vi "MarvinTester.vi"() -> ()   [LabVIEW 2017]
uses:
  <vilib>/Instr/_visa.llb/VISA Configure Serial Port (Instr).vi
panel:
  out "TX":string
  out "RX":string
  out "(hi.lo)":u32 format="%.0x"
  in  "GetOUTIO3":bool
  out "S2 GIO 19":bool
  out "S2 GIO 18":bool
  out "S2 GIO 17":bool
  out "S2 GIO 11":bool
  out "S2 GIO 3":bool
  out "S2 GIO 1":bool
  out "S1 GIO 19":bool
  out "S1 GIO 18":bool
  out "S1 GIO 17":bool
  out "S1 GIO 15":bool
  out "S1 GIO 11":bool
  out "S1 GIO 3":bool
  out "S1 GIO 1":bool
  in  "GetIO 2":bool
  out "S2 GIO 15 R":bool
  in  "Reset":bool
  in  "SetDefault":bool
  out "GetIO":u8[](array[numeric])
  out "Ver":string=" "
  in  "Get  ver":bool
  out "PWM Reading":u32
  out "Time Plot":i32=-1
  out "error out":errorcluster
  in  "stop":bool
  in  "Ring":u16(ring) items=["None", "Moment", "Get IO"]
  out "packet PWM":u8[](array[numeric])
  in  "Tab Control":enum32{"Page 3", "Page 4", "Page 2"}(tab)
  in  "GetIO2":bool
  out "out_io1":u32 format="%.0b"
  in  "SetDAC":bool
  in  "I_O":u32 format="%.0b"
  in  "ADC":bool
  in  "ADC num":u8=3
  out "out_io1 2":u32
  in  "DAC":u32
  out "x*y":dbl
  in  "GetADCTester":T1(ring)
  in  "TimeToGet":i32
  in  "Read On/Off":bool
  out "ADCValOutput Single":dbl
  in  "idx":i32
  in  "TA[idx]":bool
  in  "Disconect 2":bool
  in  "110":bool
  in  "120":bool
  in  "90":bool
  in  "60":bool
  in  "100":bool
  in  "20":bool
  in  "70":bool
  in  "40":bool
  in  "30":bool
  in  "80":bool
  in  "50":bool
  in  "10":bool
  in  "25":bool
  in  "0":bool
  in  "COM Port Marvin":refnum<visa-resource-name>="COM1"
  in  "Connect Marvin":bool
  out "CommIcon Marvin":bool=TRUE
  out "String":string
  in  "K15":bool
  in  "Firmeware":bool
  in  "K16":bool
  in  "K17":bool
  in  "Power":bool
  in  "Fan":bool
  in  "VEnable":bool
  out "CurrSp Graph":cluster{"n":dbl, "T":dbl}[](graph)
  out "Frequency":dbl
  in  "Plot On":bool
  in  "Plot OFF":bool
  in  "Get":bool
  in  "Clear":bool
  in  "Plot Time":i32=70
  out "Load":dbl
  out "String 2":string
  in  "COM Port Control":refnum<visa-resource-name>="COM1"
  in  "Time":i32=-1
  out "err tx":errorcluster
  out "Write array":u8[](array[numeric]) format="%x"
  in  "Flag Stop T":bool
  out "VISA":refnum<visa-resource-name>
  out "CommIcon":bool=TRUE
  out "Read array":u8[](array[numeric]) format="%x"
  out "Cmd Id":u8
  in  "Flag Stop I":bool=TRUE
  out "Int b":i32
  in  "Flag Stop R":bool
  out "TX":bool
  out "RX":bool
  in  "Command Menu 2":u16(ring) items=["Status", "Moment", "Isc threshold", "Vin Vout", "RESET FF", "Open", "Close", "Up Time", "Interval Period", "Nm Of Retries", "On time", "Save Parameters", "Version", "Temperature"]
  out "packet":u8[](array[numeric])
  in  "Isc1":i8
  in  "Add Unit":u8
  in  "Disconect":bool
  in  "Connect":bool
  in  "Stop VI":bool
  out "status":bool
  # "Marvin Tester"
  # "[Hz]"
  # "SW Version"
  # "ver : 00.02.a"
  # "I/O"
  # "ADC"
  # "DAC"
  # "0-4"
  # "V=ADC*3.3/4096"
  # "Term1  -0\nTerm2  -1\nCurr   - 2\nEBAYFAN -3\nTempCPU -4"
  # "b0-Rly1\nb1-Rly2\nb2-Rly3\n....\nb20-Rly20\nb21-Power"
  # "[kHz]"
  # "[N.m]"
  # "[msec]"
  # "ver 0.0.1"
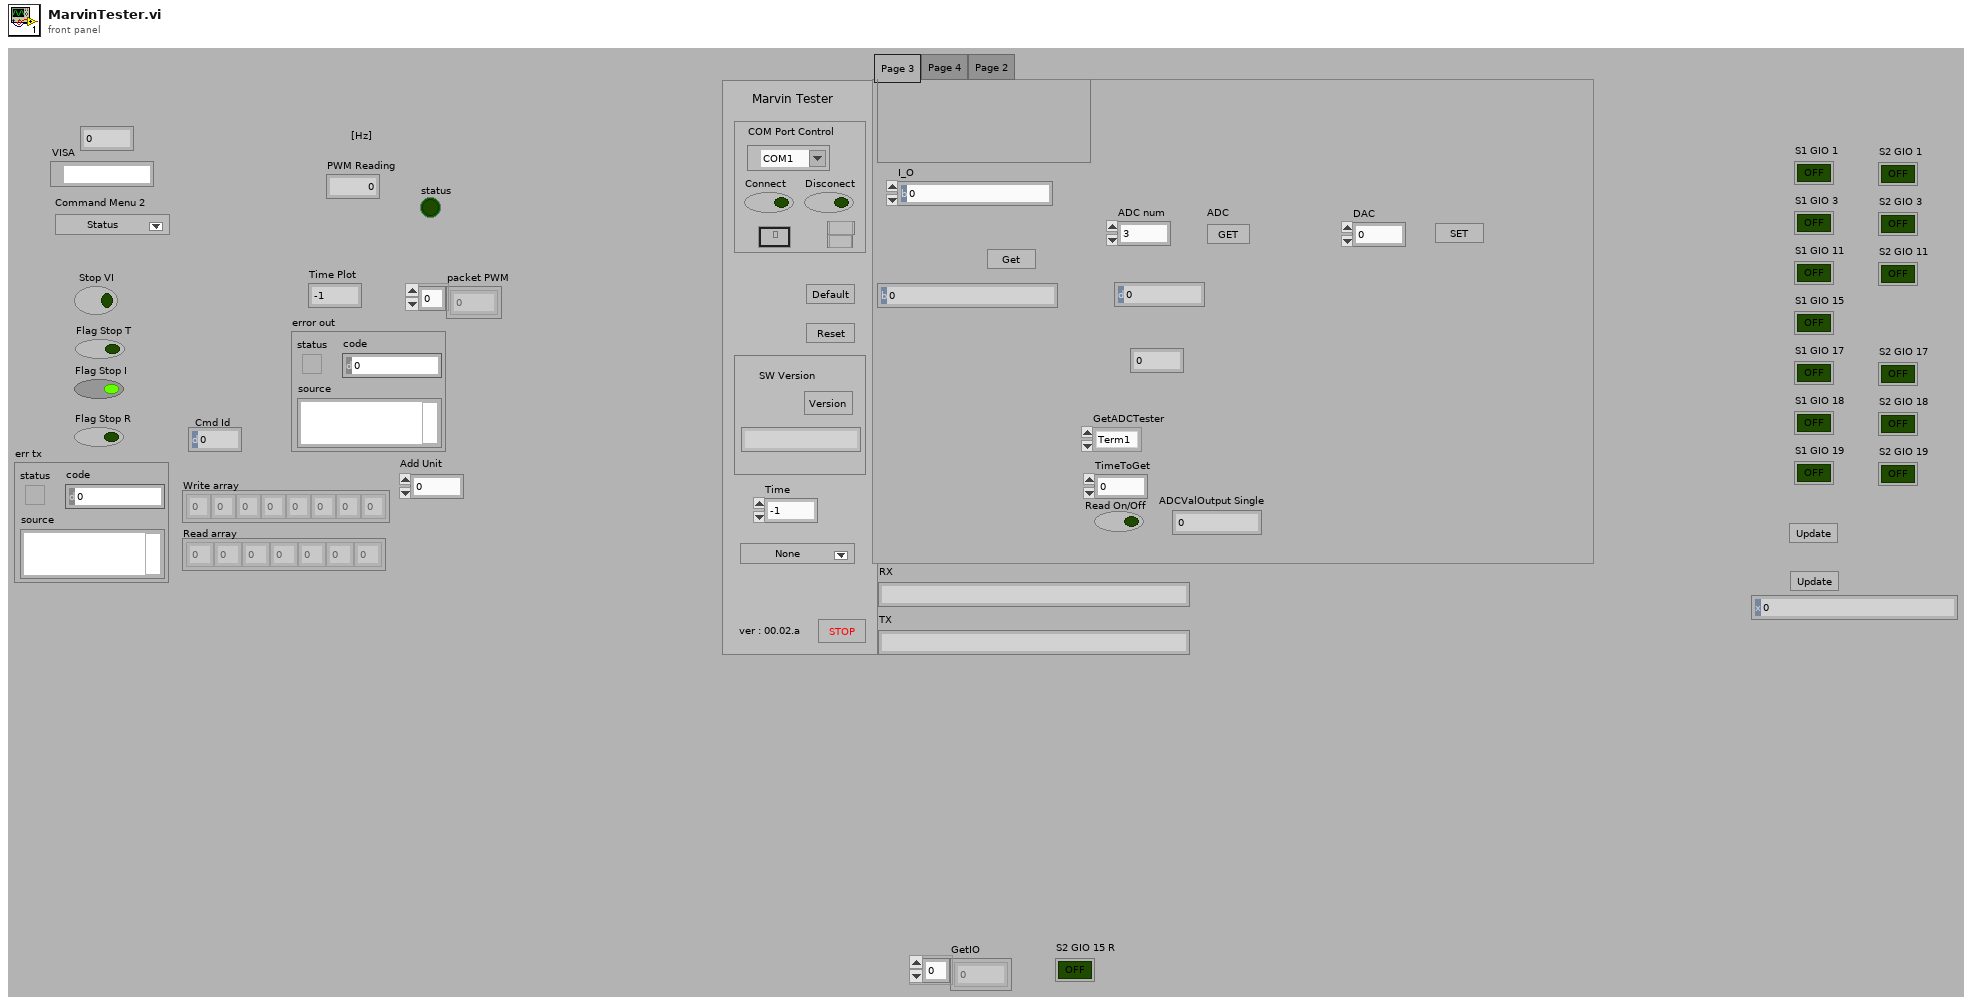
[diagram p1: front panel]
types:
  T1 = enum8{"Term1", "Term2", "Current", "Fan", "TempCPU"}
  T2 = cluster{"d1":dbl, "d2":dbl, "d3":dbl, "id":u16, "d4":dbl}
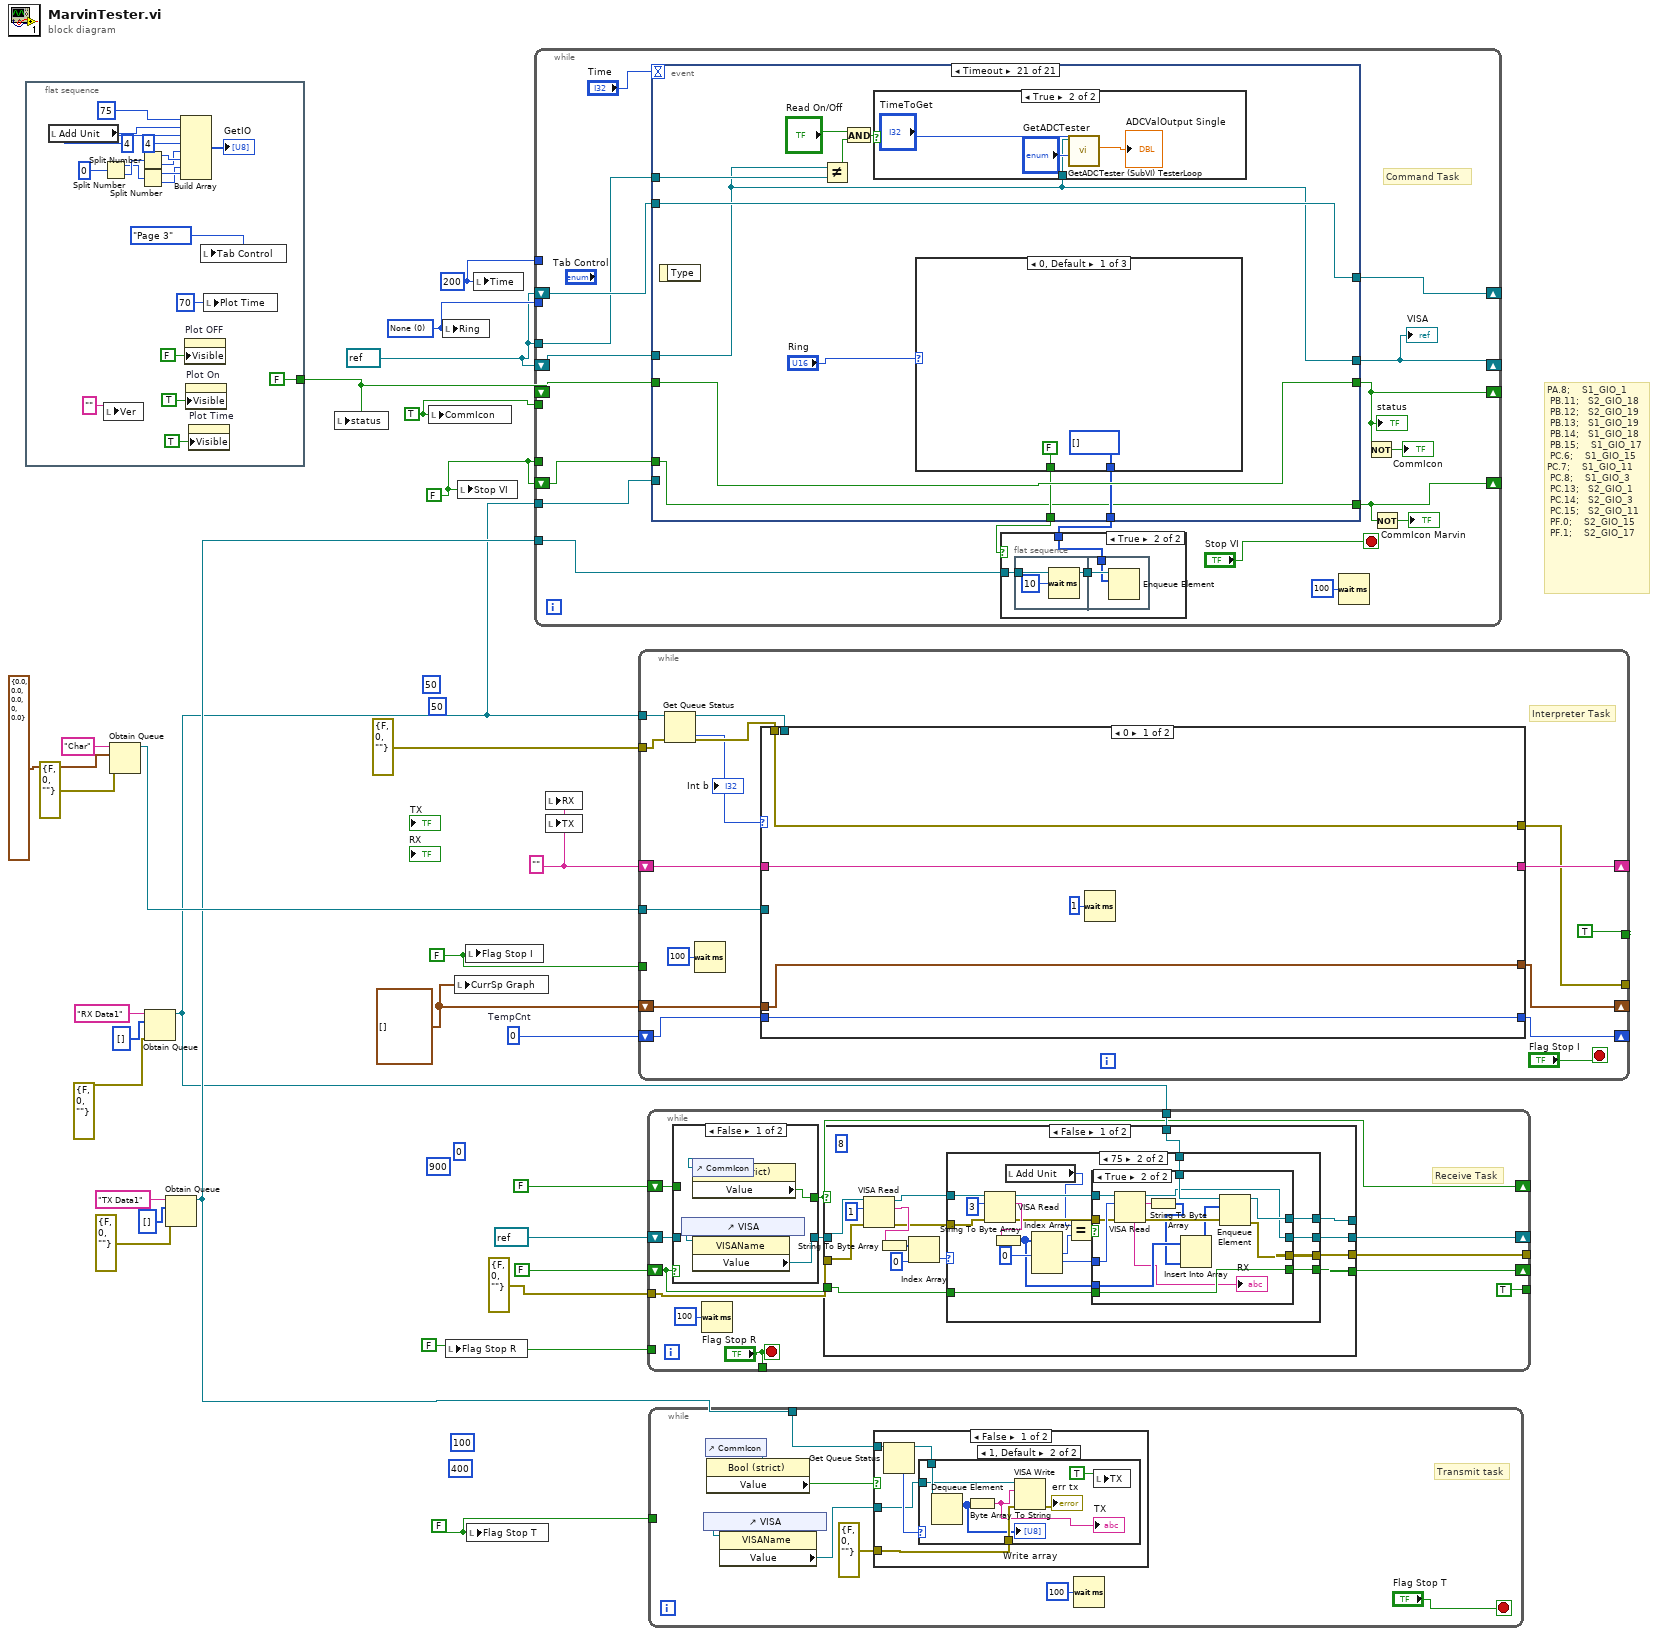
[diagram p0: block diagram]
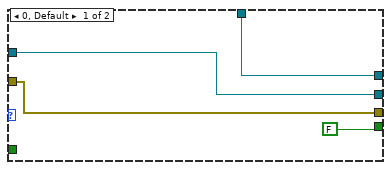
[diagram p3: hidden frame]
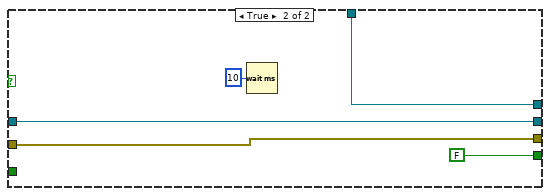
[diagram p5: hidden frame]
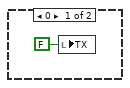
[diagram p6: hidden frame]
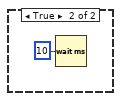
[diagram p7: hidden frame]
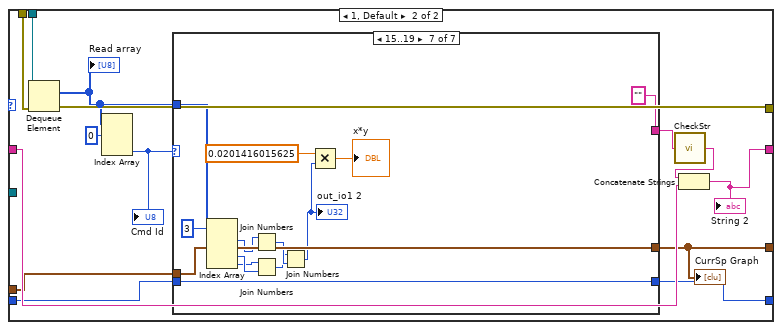
[diagram p8: hidden frame]
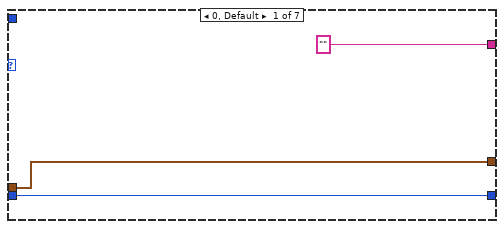
[diagram p9: hidden frame]
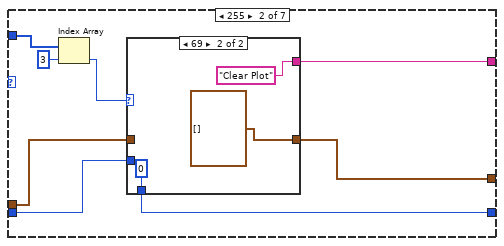
[diagram p10: hidden frame]
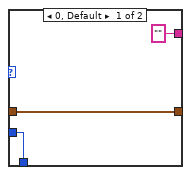
[diagram p11: hidden frame]
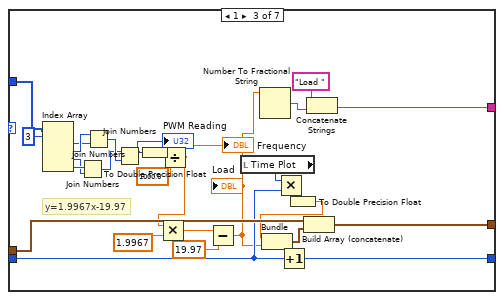
[diagram p12: hidden frame]
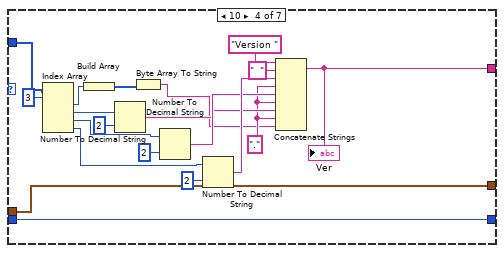
[diagram p13: hidden frame]
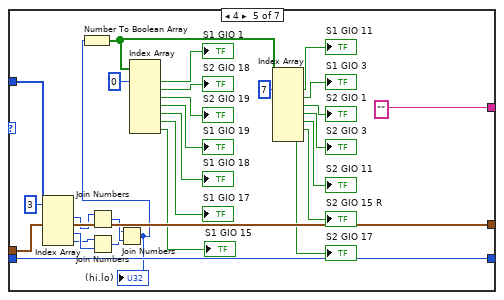
[diagram p14: hidden frame]
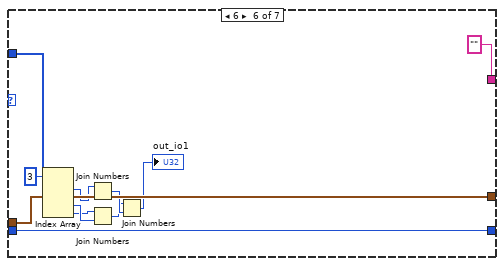
[diagram p15: hidden frame]
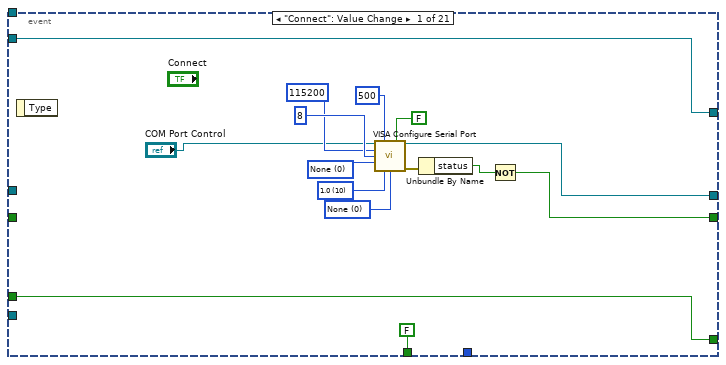
[diagram p17: hidden frame]
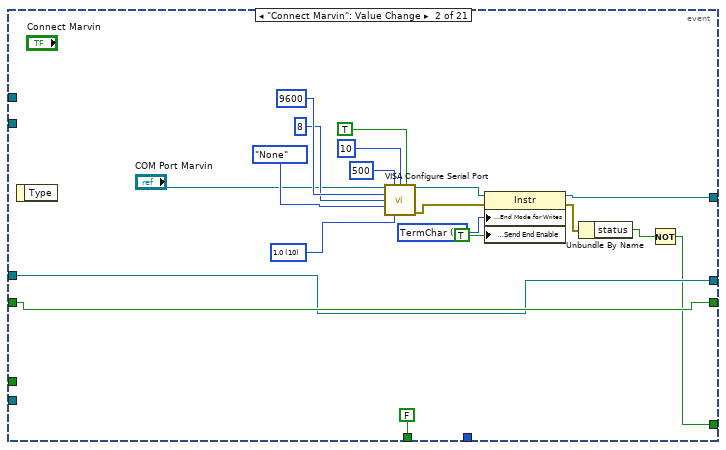
[diagram p18: hidden frame]
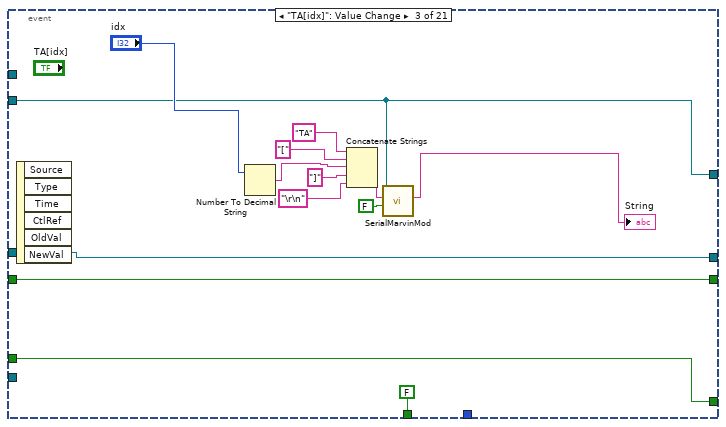
[diagram p19: hidden frame]
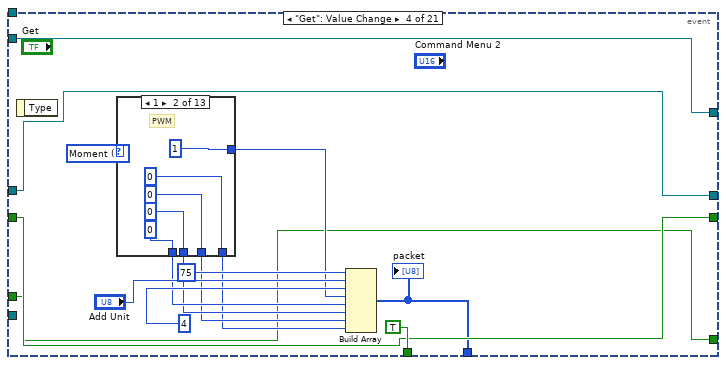
[diagram p20: hidden frame]
diagram:
  w8 = u16 0  # TempCnt
  w5 = cluster{"n":dbl, "T":dbl}[] [] ("Current Graph 4")
  w9 = 200 ("Time")
  w10 = u16 0 items=["None", "Moment"] ("Ring")
  w11 = TRUE ("CommIcon")
  w3 = FALSE
  (unwired) 400 ("Priority")
  (unwired) i64 100 ("Period")
  (unwired) i64 50 ("Period")
  (unwired) 50 ("Priority")
  (unwired) 900 ("Priority")
  (unwired) i64 0 ("Period")
  w14 = FALSE
  w2 = ""
  w28 = FALSE
  w29 = FALSE
  w1 = refnum<visa-resource-name> refnum ("VISA resource name out")
  # "PA.8;   \tS1_GIO_1\n\tPB.11;  \tS2_GIO_18\n\tPB.12;  \tS2_GIO_19\n\tPB.13;  \tS1_GIO_19\n\tPB.14;  \tS1_GIO_18\n\tPB.15;   \tS1_GIO_17\n\tPC.6;   \tS1_GIO_15\nPC.7;   \tS1_GIO_11\n\tPC.8;   \tS1_GIO_3\n\tPC.13;  \tS2_GIO_1\n\tPC.14;  \tS2_GIO_3\n\tPC.15;  \tS2_GIO_11\n\tPF.0;  \t\tS2_GIO_15\n\tPF.1;  \t\tS2_GIO_17"
  n1 = flat-sequence {
    tunnel: [FALSE] -> w7
    frame #0 {
      n2 = local read "Add Unit"() -> (w39:u8)
      n3 = Split Number(x=u32 0) -> (hi(x)=w37:u16, lo(x)=w38:u16)
      n4 = local write "Ver"("" ("Ver")) -> ()
      n5 = Split Number(x=w38) -> (hi(x)=w36:u8, lo(x)=w35:u8)
      n6 = Split Number(x=w37) -> (hi(x)=w34:u8, lo(x)=w33:u8)
      n7 = Build Array(u8 75, w39, u8 4 ("Length"), u8 4, w35, w36, w33, w34) -> (→"GetIO":u8[])
      n8 = property on="Plot OFF" class="Bool"("Visible"=FALSE) -> ()  [unwired: 2 in, 2 out]
      n9 = property on="Plot On" class="Bool"("Visible"=TRUE) -> ()  [unwired: 2 in, 2 out]
      n10 = property on="Plot Time" class="DigNum (strict)"("Visible"=TRUE) -> ()  [unwired: 2 in, 2 out]
      n11 = local write "Tab Control"(enum32{"Page 3", "Page 4", "Page 2"}."Page 3" ("Tab Control")) -> ()
      n12 = local write "Plot Time"(70 ("Plot Time")) -> ()
    }
  }
  n13 = Obtain Queue(name (unnamed)="Char", element data type=T2 {"d1"=0.0, "d2"=0.0, "d3"=0.0, "id"=0, "d4"=0.0}, error in (no error)=errorcluster {"status"=FALSE, "code"=0, "source"=""}) -> (queue out=w19:refnum<queue>)  [unwired: 2 in, 2 out]
  n14 = Obtain Queue(name (unnamed)="RX Data1", element data type=u8[] [], error in (no error)=errorcluster {"status"=FALSE, "code"=0, "source"=""}) -> (queue out=w6:refnum<queue>)  [unwired: 2 in, 2 out]
  n15 = Obtain Queue(name (unnamed)="TX Data1", element data type=u8[] [], error in (no error)=errorcluster {"status"=FALSE, "code"=0, "source"=""}) -> (queue out=w13:refnum<queue>)  [unwired: 2 in, 2 out]
  n16 = local write "status"(w7) -> ()
  n17 = local write "CommIcon"(w11) -> ()
  n18 = local write "Ring"(w10) -> ()
  n19 = local write "Flag Stop R"(w29) -> ()
  n20 = local write "CurrSp Graph"(w5) -> ()
  n21 = local write "Stop VI"(w3) -> ()
  n22 = local write "Flag Stop I"(w28) -> ()
  n23 = local write "Flag Stop T"(w14) -> ()
  n24 = local write "Time"(w9) -> ()
  n25 = while {
    shift-right: [w59] -> _
    shift-left: w1 -> [w66]
    shift-right: [w58] -> _
    shift-left: w7 -> [w65]
    tunnel: w13 -> [w61]
    tunnel: w3 -> [_]
    tunnel: w11 -> [_]
    tunnel: w10 -> [_]
    tunnel: w9 -> [_]
    tunnel: w6 -> [w56]
    shift-right: [w54] -> _
    shift-left: w1 -> [w53]
    shift-right: [w52] -> _
    shift-left: w3 -> [w51]
    tunnel: w1 -> [w50]
    stop <- "Stop VI" stop-if-true
    # "Command Task"
    n26 = event shown="[20] Timeout" {
      selector: _ -> [_ _ _ _ _ _ _ _ _ _ _ _ _ _ _ _ _ _ _ _ _]
      dyn-events: _ -> [_ _ _ _ _ _ _ _ _ _ _ _ _ _ _ _ _ _ _ _ _]
      timeout: "Time" -> [_ _ _ _ _ _ _ _ _ _ _ _ _ _ _ _ _ _ _ _ _]
      tunnel: [w82 w105 w111 w126 w208 w286 w317 w594 w605 w622 w639 w656 w673 w690 w719 w729 w736 w740 refnum<visa-resource-name> refnum ("VISA resource name out") w755 w759] -> w59
      tunnel: w66 -> [_ w105 w111 w126 w208 w286 w317 w594 w605 w622 w639 w656 w673 w690 w719 w729 w736 w740 w751 w755 w759]
      tunnel: [w80 w106 w110 w125 w207 w296 w316 w597 w613 w630 w647 w664 w681 w698 w721 w731 w738 FALSE FALSE w753 w768] -> w58
      tunnel: w65 -> [_ w106 w110 w125 w207 w296 w316 w597 w613 w630 w647 w664 w681 w698 w721 w731 w738 _ _ w753 w768]
      tunnel: [_ _ _ w124 w206 w295 w319 w596 w603 w620 w637 w654 w671 w688 _ _ _ _ _ _ w766] -> w60
      tunnel: [FALSE FALSE FALSE TRUE TRUE TRUE TRUE TRUE TRUE TRUE TRUE TRUE TRUE TRUE FALSE FALSE FALSE FALSE FALSE FALSE w767] -> w62
      tunnel: w56 -> [_ _ _ _ _ _ _ _ _ _ _ _ _ _ _ _ w735 _ _ _ _]
      tunnel: [w75 w92 w112 w123 w203 w284 w315 w589 w602 w619 w636 w653 w670 w687 w704 w723 w733 w741 w747 refnum<visa-resource-name> refnum ("VISA resource name out") w764] -> w54
      tunnel: w53 -> [w75 _ w112 w123 w203 w284 w315 w589 w602 w619 w636 w653 w670 w687 w704 w723 w733 w741 w747 w754 w764]
      tunnel: [w74 w89 w108 w122 w202 w283 w314 w588 w601 w618 w635 w652 w669 w686 w703 w722 w732 w739 w746 FALSE w763] -> w52
      tunnel: w51 -> [w74 _ w108 w122 w202 w283 w314 w588 w601 w618 w635 w652 w669 w686 w703 w722 w732 w739 w746 _ w763]
      tunnel: w50 -> [_ _ _ _ _ _ _ _ _ _ _ _ _ _ _ _ _ _ _ _ w760]
      event "Connect": Value Change {
        w88 = u16 0 items=["None"=0, "XON/XOFF"=1, "RTS/CTS"=2, "DTR/DSR"=4] ("flow control")
        w87 = u16 10 items=["1.0"=10, "1.5"=15, "2.0"=20] ("stop bits")
        w86 = u16 0 items=["None", "Odd", "Even", "Mark", "Space"] ("parity")
        n27 = event-data() -> ()  [unwired: 1 in, 1 out]
        n28 = call-poly "VISA Configure Serial Port"("VISA resource name"="COM Port Control", "timeout (10sec)"=u32 500, "Enable Termination\nChar (T)"=FALSE ("Enable Termination\nChar (T)"), "baud rate (9600)"=u32 115200 ("baud rate"), "data bits (8)"=u16 8 ("data bits"), "parity (0:none)"=w86, "stop bits (10: 1 bit)"=w87, "flow control (0:none)"=w88) -> ("VISA resource name out"=w82:refnum<visa-resource-name>, "error out"=w79:errorcluster)  [unwired: 6 in]
        n29 = Unbundle By Name(w79) -> ("status"=w81:bool)
        n30 = Not(x=w81) -> (.not. x?=w80:bool)
      }
      event "Connect Marvin": Value Change {
        w104 = u16 2 items=["None", "LastBit", "TermChar", "Break"] ("Serial Settings:Serial End Mode for Writes")
        w97 = u16 10 items=["1.0"=10, "1.5"=15, "2.0"=20] ("stop bits (10: 1 bit)")
        n31 = event-data() -> ()  [unwired: 1 in, 1 out]
        n32 = call-poly "VISA Configure Serial Port"("VISA resource name"="COM Port Marvin", "timeout (10sec)"=u32 500, "termination char\n(0xA = '\\n' = LF)"=u8 10 ("termination char\n(0xA = '\\n' = LF)"), "Enable Termination\nChar (T)"=TRUE ("Enable Termination\nChar (T)"), "baud rate (9600)"=u32 9600, "data bits (8)"=u16 8, "parity (0:none)"=enum16{"None", "Odd", "Even", "Mark", "Space"}."None", "stop bits (10: 1 bit)"=w97) -> ("VISA resource name out"=w95:refnum<visa-resource-name>, "error out"=w94:errorcluster)  [unwired: 6 in]
        n33 = property class="Instr"(reference=w95, error in=w94, "Serial Settings:End Mode for Writes"=w104, "Message Based Settings:Send End Enable"=TRUE) -> (reference out=w92:refnum<visa-resource-name>, error out=w90:errorcluster)
        n34 = Unbundle By Name(w90) -> ("status"=w91:bool)
        n35 = Not(x=w91) -> (.not. x?=w89:bool)
      }
      event "TA[idx]": Value Change {
        n36 = event-data() -> ()  [unwired: 1 in, 6 out]
        n37 = Number To Decimal String(number="idx") -> (decimal integer string=w115:string)  [unwired: 1 in]
        n38 = Concatenate Strings("TA" ("string"), "[", w115, "]", "\r\n" ("write buffer")) -> (w116:string)
        n39 = call "SerialMarvinMod.vi"("Clear Log"=FALSE, "write buffer"=w116, "VISA resource name"=w112) -> ("read buffer"=→"String":string)  [unwired: 7 in, 1 out]
      }
      event "Get": Value Change {
        w128 = u16 1 items=["Status", "Moment", "Isc threshold", "Vin Vout", "RESET FF", "Open", "Close", "Up Time", "Interval Period", "Nm Of Retries", "On time", "Save Parameters", "Version", "Temperature"] ("Command Menu 3")
        n40 = event-data() -> ()  [unwired: 1 in, 1 out]
        n41 = case shown="1" w128 {
          tunnel: [u8 0 u8 1 u8 2 u8 15 u8 4 u8 4 u8 5 u8 6 u8 7 u8 8 u8 9 u8 10 u8 16] -> w133
          tunnel: [u8 0 u8 0 u8 0 u8 0 u8 0 u8 0 u8 0 u8 0 u8 0 u8 0 u8 0 u8 0 u8 0] -> w131
          tunnel: [u8 0 u8 0 u8 0 u8 0 u8 0 u8 0 u8 0 u8 0 u8 0 u8 0 u8 0 u8 0 u8 0] -> w130
          tunnel: [u8 0 u8 0 "Isc1" u8 0 u8 1 u8 0 u8 0 u8 0 u8 0 u8 0 u8 0 u8 0 u8 0] -> w132
          tunnel: [u8 0 u8 0 u8 0 u8 0 u8 0 u8 0 u8 0 u8 0 u8 0 u8 0 u8 0 u8 0 u8 0] -> w129
          frame 0, Default {
            # "Status"
          }
          frame 1 {
            # "PWM"
          }
          frame 2 {
          }
          frame 3 {
            # "Vout"
          }
          frame 5 {
          }
          frame 6 {
          }
          frame 7 {
          }
          frame 8 {
          }
          frame 9 {
          }
          frame 10 {
          }
          frame 11 {
          }
          frame 12 {
          }
          frame 13 {
          }
        }
        n42 = Build Array(u8 75, "Add Unit", u8 4 ("Length"), w133, w132, w131, w130, w129) -> (w124:u8[])
        "packet" <- w124
      }
      event "Get  ver": Value Change {
        w210 = u16 12 items=["Status", "Moment", "Isc threshold", "Vin Vout", "RESET FF", "Open", "Close", "Up Time", "Interval Period", "Nm Of Retries", "On time", "Save Parameters", "Version", "Temperature"] ("Command Menu 3")
        n43 = event-data() -> ()  [unwired: 1 in, 1 out]
        n44 = local read "Add Unit"() -> (w205:u8)
        n45 = case shown="0, Default" w210 {
          tunnel: [u8 0 u8 1 u8 2 u8 15 u8 4 u8 4 u8 5 u8 6 u8 7 u8 8 u8 9 u8 10 u8 16] -> w215
          tunnel: [u8 0 u8 0 u8 0 u8 0 u8 0 u8 0 u8 0 u8 0 u8 0 u8 0 u8 0 u8 0 u8 0] -> w213
          tunnel: [u8 0 u8 0 u8 0 u8 0 u8 0 u8 0 u8 0 u8 0 u8 0 u8 0 u8 0 u8 0 u8 0] -> w212
          tunnel: [u8 0 u8 0 u8 0 u8 0 u8 1 u8 0 u8 0 u8 0 u8 0 u8 0 u8 0 u8 0 u8 0] -> w214
          tunnel: [u8 0 u8 0 u8 0 u8 0 u8 0 u8 0 u8 0 u8 0 u8 0 u8 0 u8 0 u8 0 u8 0] -> w211
          frame 0, Default {
            # "Status"
          }
          frame 1 {
            # "PWM"
          }
          frame 2 {
          }
          frame 3 {
            # "Vout"
          }
          frame 5 {
          }
          frame 6 {
          }
          frame 7 {
          }
          frame 8 {
          }
          frame 9 {
          }
          frame 10 {
          }
          frame 11 {
          }
          frame 12 {
          }
          frame 13 {
          }
        }
        n46 = local write "Ver"("" ("Ver")) -> ()
        n47 = Build Array(u8 75, w205, u8 4 ("Length"), w215, w214, w213, w212, w211) -> (w206:u8[])
      }
      event "I_O": Value Change {
        n48 = event-data() -> ()  [unwired: 1 in, 3 out]
        n49 = local read "Add Unit"() -> (w294:u8)
        n50 = To Unsigned Long Integer(number="I_O") -> (unsigned 32bit integer=w287:u32)
        n51 = Split Number(x=w287) -> (hi(x)=w292:u16, lo(x)=w293:u16)
        n52 = Split Number(x=w293) -> (hi(x)=w291:u8, lo(x)=w290:u8)
        n53 = Split Number(x=w292) -> (hi(x)=w289:u8, lo(x)=w288:u8)
        n54 = Build Array(u8 75, w294, u8 4 ("Length"), u8 2, w290, w291, w288, w289) -> (w295:u8[])
      }
      event "0", "25", "10", "50", "80", "30", "40", "70", "20", "100", "60", "90", "120", "110", "K15", "Firmeware", "K16", "K17", "Power", "Fan", "VEnable": Value Change {
        n55 = event-data() -> ("CtlRef"=w322:refnum<vi>, "NewVal"=w320:bool)  [unwired: 1 in, 1 out]
        n56 = property class="Bool (strict)"(reference=w322) -> ("Label.Text"=w321:string)  [unwired: 1 in, 2 out]
        n57 = Build Array("K15", "K16", "K17", "VEnable", "Firmeware", "Fan", "Power") -> (w302:bool[])
        n58 = Initialize Array(FALSE, 14 ("dimension size")) -> (w303:bool[])
        n59 = Build Array (concatenate)(w303, w302) -> (w301:bool[])
        n60 = Boolean Array To Number(Boolean array=w301) -> (number=w306:u32)
        n61 = case shown="\"120\"" w321 {
          tunnel: w320 -> [w330 w348 w365 w383 w400 w418 w436 w455 w473 w490 w509 w526 w544 w562 _]
          tunnel: [w327 w345 w362 w380 w397 w415 w433 w452 w470 w487 w506 w523 w541 w559 w575] -> w319
          tunnel: w306 -> [w324 w343 w359 w378 w395 w413 w431 w450 w469 w485 w504 w521 w539 w557 w576]
          frame "0" {
            n62 = Select(t=u32 1 ("number"), s=w330, f=u32 0) -> (s? t:f=w328:u32)
            n63 = local read "Add Unit"() -> (w331:u8)
            n64 = To Unsigned Long Integer(number=w328) -> (unsigned 32bit integer=w325:u32)
            n65 = Or(x=w324, y=w325) -> (x .or. y?=w323:u32)
            n66 = Split Number(x=w323) -> (hi(x)=w336:u16, lo(x)=w337:u16)
            n67 = Split Number(x=w337) -> (hi(x)=w335:u8, lo(x)=w334:u8)
            n68 = Split Number(x=w336) -> (hi(x)=w333:u8, lo(x)=w332:u8)
            n69 = Build Array(u8 75, w331, u8 4 ("Length"), u8 2, w334, w335, w332, w333) -> (w327:u8[])
          }
          frame "10" {
            n70 = Select(t=u32 2 ("number"), s=w348, f=u32 0) -> (s? t:f=w346:u32)
            n71 = local read "Add Unit"() -> (w349:u8)
            n72 = To Unsigned Long Integer(number=w346) -> (unsigned 32bit integer=w342:u32)
            n73 = Or(x=w343, y=w342) -> (x .or. y?=w341:u32)
            n74 = Split Number(x=w341) -> (hi(x)=w354:u16, lo(x)=w355:u16)
            n75 = Split Number(x=w355) -> (hi(x)=w353:u8, lo(x)=w352:u8)
            n76 = Split Number(x=w354) -> (hi(x)=w351:u8, lo(x)=w350:u8)
            n77 = Build Array(u8 75, w349, u8 4 ("Length"), u8 2, w352, w353, w350, w351) -> (w345:u8[])
          }
          frame "20" {
            n78 = Select(t=u32 4 ("number"), s=w365, f=u32 0) -> (s? t:f=w363:u32)
            n79 = local read "Add Unit"() -> (w367:u8)
            n80 = To Unsigned Long Integer(number=w363) -> (unsigned 32bit integer=w361:u32)
            n81 = Or(x=w359, y=w361) -> (x .or. y?=w360:u32)
            n82 = Split Number(x=w360) -> (hi(x)=w372:u16, lo(x)=w373:u16)
            n83 = Split Number(x=w373) -> (hi(x)=w371:u8, lo(x)=w370:u8)
            n84 = Split Number(x=w372) -> (hi(x)=w369:u8, lo(x)=w368:u8)
            n85 = Build Array(u8 75, w367, u8 4 ("Length"), u8 2, w370, w371, w368, w369) -> (w362:u8[])
          }
          frame "25" {
            n86 = Select(t=u32 8 ("number"), s=w383, f=u32 0) -> (s? t:f=w381:u32)
            n87 = local read "Add Unit"() -> (w385:u8)
            n88 = To Unsigned Long Integer(number=w381) -> (unsigned 32bit integer=w379:u32)
            n89 = Or(x=w378, y=w379) -> (x .or. y?=w377:u32)
            n90 = Split Number(x=w377) -> (hi(x)=w390:u16, lo(x)=w391:u16)
            n91 = Split Number(x=w391) -> (hi(x)=w389:u8, lo(x)=w388:u8)
            n92 = Split Number(x=w390) -> (hi(x)=w387:u8, lo(x)=w386:u8)
            n93 = Build Array(u8 75, w385, u8 4 ("Length"), u8 2, w388, w389, w386, w387) -> (w380:u8[])
          }
          frame "30" {
            n94 = Select(t=u32 16 ("number"), s=w400, f=u32 0) -> (s? t:f=w398:u32)
            n95 = local read "Add Unit"() -> (w402:u8)
            n96 = To Unsigned Long Integer(number=w398) -> (unsigned 32bit integer=w403:u32)
            n97 = Or(x=w403, y=w395) -> (x .or. y?=w396:u32)
            n98 = Split Number(x=w396) -> (hi(x)=w408:u16, lo(x)=w409:u16)
            n99 = Split Number(x=w409) -> (hi(x)=w407:u8, lo(x)=w406:u8)
            n100 = Split Number(x=w408) -> (hi(x)=w405:u8, lo(x)=w404:u8)
            n101 = Build Array(u8 75, w402, u8 4 ("Length"), u8 2, w406, w407, w404, w405) -> (w397:u8[])
          }
          frame "40" {
            n102 = Select(t=u32 32 ("number"), s=w418, f=u32 0) -> (s? t:f=w416:u32)
            n103 = local read "Add Unit"() -> (w420:u8)
            n104 = To Unsigned Long Integer(number=w416) -> (unsigned 32bit integer=w421:u32)
            n105 = Or(x=w413, y=w421) -> (x .or. y?=w414:u32)
            n106 = Split Number(x=w414) -> (hi(x)=w426:u16, lo(x)=w427:u16)
            n107 = Split Number(x=w427) -> (hi(x)=w425:u8, lo(x)=w424:u8)
            n108 = Split Number(x=w426) -> (hi(x)=w423:u8, lo(x)=w422:u8)
            n109 = Build Array(u8 75, w420, u8 4 ("Length"), u8 2, w424, w425, w422, w423) -> (w415:u8[])
          }
          frame "50" {
            n110 = Select(t=u32 64 ("number"), s=w436, f=u32 0) -> (s? t:f=w434:u32)
            n111 = local read "Add Unit"() -> (w438:u8)
            n112 = To Unsigned Long Integer(number=w434) -> (unsigned 32bit integer=w439:u32)
            n113 = Or(x=w431, y=w439) -> (x .or. y?=w432:u32)
            n114 = Split Number(x=w432) -> (hi(x)=w444:u16, lo(x)=w445:u16)
            n115 = Split Number(x=w445) -> (hi(x)=w443:u8, lo(x)=w442:u8)
            n116 = Split Number(x=w444) -> (hi(x)=w441:u8, lo(x)=w440:u8)
            n117 = Build Array(u8 75, w438, u8 4 ("Length"), u8 2, w442, w443, w440, w441) -> (w433:u8[])
          }
          frame "60" {
            n118 = Select(t=u32 128 ("number"), s=w455, f=u32 0) -> (s? t:f=w453:u32)
            n119 = local read "Add Unit"() -> (w457:u8)
            n120 = To Unsigned Long Integer(number=w453) -> (unsigned 32bit integer=w451:u32)
            n121 = Or(x=w450, y=w451) -> (x .or. y?=w449:u32)
            n122 = Split Number(x=w449) -> (hi(x)=w462:u16, lo(x)=w463:u16)
            n123 = Split Number(x=w463) -> (hi(x)=w461:u8, lo(x)=w460:u8)
            n124 = Split Number(x=w462) -> (hi(x)=w459:u8, lo(x)=w458:u8)
            n125 = Build Array(u8 75, w457, u8 4 ("Length"), u8 2, w460, w461, w458, w459) -> (w452:u8[])
          }
          frame "70" {
            n126 = Select(t=u32 256 ("number"), s=w473, f=u32 0) -> (s? t:f=w471:u32)
            n127 = local read "Add Unit"() -> (w475:u8)
            n128 = To Unsigned Long Integer(number=w471) -> (unsigned 32bit integer=w468:u32)
            n129 = Or(x=w469, y=w468) -> (x .or. y?=w467:u32)
            n130 = Split Number(x=w467) -> (hi(x)=w480:u16, lo(x)=w481:u16)
            n131 = Split Number(x=w481) -> (hi(x)=w479:u8, lo(x)=w478:u8)
            n132 = Split Number(x=w480) -> (hi(x)=w477:u8, lo(x)=w476:u8)
            n133 = Build Array(u8 75, w475, u8 4 ("Length"), u8 2, w478, w479, w476, w477) -> (w470:u8[])
          }
          frame "80" {
            n134 = Select(t=u32 512 ("number"), s=w490, f=u32 0) -> (s? t:f=w488:u32)
            n135 = local read "Add Unit"() -> (w492:u8)
            n136 = To Unsigned Long Integer(number=w488) -> (unsigned 32bit integer=w493:u32)
            n137 = Or(x=w485, y=w493) -> (x .or. y?=w486:u32)
            n138 = Split Number(x=w486) -> (hi(x)=w498:u16, lo(x)=w499:u16)
            n139 = Split Number(x=w499) -> (hi(x)=w497:u8, lo(x)=w496:u8)
            n140 = Split Number(x=w498) -> (hi(x)=w495:u8, lo(x)=w494:u8)
            n141 = Build Array(u8 75, w492, u8 4 ("Length"), u8 2, w496, w497, w494, w495) -> (w487:u8[])
          }
          frame "90" {
            n142 = Select(t=u32 1024 ("number"), s=w509, f=u32 0) -> (s? t:f=w507:u32)
            n143 = local read "Add Unit"() -> (w511:u8)
            n144 = To Unsigned Long Integer(number=w507) -> (unsigned 32bit integer=w505:u32)
            n145 = Or(x=w504, y=w505) -> (x .or. y?=w503:u32)
            n146 = Split Number(x=w503) -> (hi(x)=w516:u16, lo(x)=w517:u16)
            n147 = Split Number(x=w517) -> (hi(x)=w515:u8, lo(x)=w514:u8)
            n148 = Split Number(x=w516) -> (hi(x)=w513:u8, lo(x)=w512:u8)
            n149 = Build Array(u8 75, w511, u8 4 ("Length"), u8 2, w514, w515, w512, w513) -> (w506:u8[])
          }
          frame "100" {
            n150 = Select(t=u32 2048 ("number"), s=w526, f=u32 0) -> (s? t:f=w524:u32)
            n151 = local read "Add Unit"() -> (w528:u8)
            n152 = To Unsigned Long Integer(number=w524) -> (unsigned 32bit integer=w529:u32)
            n153 = Or(x=w521, y=w529) -> (x .or. y?=w522:u32)
            n154 = Split Number(x=w522) -> (hi(x)=w534:u16, lo(x)=w535:u16)
            n155 = Split Number(x=w535) -> (hi(x)=w533:u8, lo(x)=w532:u8)
            n156 = Split Number(x=w534) -> (hi(x)=w531:u8, lo(x)=w530:u8)
            n157 = Build Array(u8 75, w528, u8 4 ("Length"), u8 2, w532, w533, w530, w531) -> (w523:u8[])
          }
          frame "110" {
            n158 = local read "Add Unit"() -> (w546:u8)
            n159 = Select(t=u32 4096 ("number"), s=w544, f=u32 0) -> (s? t:f=w542:u32)
            n160 = To Unsigned Long Integer(number=w542) -> (unsigned 32bit integer=w547:u32)
            n161 = Or(x=w539, y=w547) -> (x .or. y?=w540:u32)
            n162 = Split Number(x=w540) -> (hi(x)=w552:u16, lo(x)=w553:u16)
            n163 = Split Number(x=w553) -> (hi(x)=w551:u8, lo(x)=w550:u8)
            n164 = Split Number(x=w552) -> (hi(x)=w549:u8, lo(x)=w548:u8)
            n165 = Build Array(u8 75, w546, u8 4 ("Length"), u8 2, w550, w551, w548, w549) -> (w541:u8[])
          }
          frame "120" {
            n166 = Select(t=u32 8192 ("number"), s=w562, f=u32 0) -> (s? t:f=w560:u32)
            n167 = local read "Add Unit"() -> (w564:u8)
            n168 = To Unsigned Long Integer(number=w560) -> (unsigned 32bit integer=w565:u32)
            n169 = Or(x=w565, y=w557) -> (x .or. y?=w558:u32)
            n170 = Split Number(x=w558) -> (hi(x)=w570:u16, lo(x)=w571:u16)
            n171 = Split Number(x=w571) -> (hi(x)=w569:u8, lo(x)=w568:u8)
            n172 = Split Number(x=w570) -> (hi(x)=w567:u8, lo(x)=w566:u8)
            n173 = Build Array(u8 75, w564, u8 4 ("Length"), u8 2, w568, w569, w566, w567) -> (w559:u8[])
          }
          frame Default {
            n174 = local read "Add Unit"() -> (w577:u8)
            n175 = To Unsigned Long Integer(number=w576) -> (unsigned 32bit integer=w578:u32)
            n176 = Split Number(x=w578) -> (hi(x)=w583:u16, lo(x)=w584:u16)
            n177 = Split Number(x=w584) -> (hi(x)=w582:u8, lo(x)=w581:u8)
            n178 = Split Number(x=w583) -> (hi(x)=w580:u8, lo(x)=w579:u8)
            n179 = Build Array(u8 75, w577, u8 4 ("Length"), u8 2, w581, w582, w579, w580) -> (w575:u8[])
          }
        }
      }
      event "ADC": Value Change {
        w590 = u8 0 ("element")
        n180 = event-data() -> ()  [unwired: 1 in, 3 out]
        n181 = local read "Add Unit"() -> (w595:u8)
        n182 = Add(x="ADC num", y=u8 15) -> (x+y=w592:u8)
        n183 = Build Array(u8 75, w595, u8 4 ("Length"), w592, w590, w590, w590, w590) -> (w596:u8[])
      }
      event "GetIO 2": Value Change {
        n184 = event-data() -> ()  [unwired: 1 in, 1 out]
        n185 = local read "Add Unit"() -> (w612:u8)
        n186 = Split Number(x=u32 0) -> (hi(x)=w610:u16, lo(x)=w611:u16)
        n187 = Split Number(x=w611) -> (hi(x)=w609:u8, lo(x)=w608:u8)
        n188 = Split Number(x=w610) -> (hi(x)=w607:u8, lo(x)=w606:u8)
        n189 = Build Array(u8 75, w612, u8 4 ("Length"), u8 4, w608, w609, w606, w607) -> (w603:u8[])
        n190 = local write "GetIO"(w603) -> ()
      }
      event "SetDefault": Value Change {
        n191 = event-data() -> ()  [unwired: 1 in, 1 out]
        n192 = local read "Add Unit"() -> (w629:u8)
        n193 = Split Number(x=u32 0) -> (hi(x)=w627:u16, lo(x)=w628:u16)
        n194 = Split Number(x=w628) -> (hi(x)=w626:u8, lo(x)=w625:u8)
        n195 = Split Number(x=w627) -> (hi(x)=w624:u8, lo(x)=w623:u8)
        n196 = Build Array(u8 75, w629, u8 4 ("Length"), u8 9, w625, w626, w623, w624) -> (w620:u8[])
        n197 = local write "GetIO"(w620) -> ()
      }
      event "Reset": Value Change {
        n198 = event-data() -> ()  [unwired: 1 in, 1 out]
        n199 = local read "Add Unit"() -> (w646:u8)
        n200 = Split Number(x=u32 0) -> (hi(x)=w644:u16, lo(x)=w645:u16)
        n201 = Split Number(x=w645) -> (hi(x)=w643:u8, lo(x)=w642:u8)
        n202 = Split Number(x=w644) -> (hi(x)=w641:u8, lo(x)=w640:u8)
        n203 = Build Array(u8 75, w646, u8 4 ("Length"), u8 11, w642, w643, w640, w641) -> (w637:u8[])
        n204 = local write "GetIO"(w637) -> ()
      }
      event "GetIO2": Value Change {
        n205 = event-data() -> ()  [unwired: 1 in, 1 out]
        n206 = local read "Add Unit"() -> (w663:u8)
        n207 = Split Number(x=u32 0) -> (hi(x)=w661:u16, lo(x)=w662:u16)
        n208 = Split Number(x=w662) -> (hi(x)=w660:u8, lo(x)=w659:u8)
        n209 = Split Number(x=w661) -> (hi(x)=w658:u8, lo(x)=w657:u8)
        n210 = Build Array(u8 75, w663, u8 4 ("Length"), u8 6, w659, w660, w657, w658) -> (w654:u8[])
      }
      event "SetDAC": Value Change {
        n211 = event-data() -> ()  [unwired: 1 in, 1 out]
        n212 = local read "Add Unit"() -> (w680:u8)
        n213 = Split Number(x="DAC") -> (hi(x)=w678:u16, lo(x)=w679:u16)
        n214 = Split Number(x=w679) -> (hi(x)=w677:u8, lo(x)=w676:u8)
        n215 = Split Number(x=w678) -> (hi(x)=w675:u8, lo(x)=w674:u8)
        n216 = Build Array(u8 75, w680, u8 4 ("Length"), u8 7, w676, w677, w674, w675) -> (w671:u8[])
      }
      event "GetOUTIO3": Value Change {
        n217 = event-data() -> ()  [unwired: 1 in, 1 out]
        n218 = local read "Add Unit"() -> (w697:u8)
        n219 = Split Number(x=u32 0) -> (hi(x)=w695:u16, lo(x)=w696:u16)
        n220 = Split Number(x=w696) -> (hi(x)=w694:u8, lo(x)=w693:u8)
        n221 = Split Number(x=w695) -> (hi(x)=w692:u8, lo(x)=w691:u8)
        n222 = Build Array(u8 75, w697, u8 4 ("Length"), u8 8, w693, w694, w691, w692) -> (w688:u8[])
      }
      event "Plot On": Value Change {
        w709 = u16 1 items=["None", "Moment"] ("Ring")
        n223 = event-data() -> ()  [unwired: 1 in, 1 out]
        n224 = local read "Add Unit"() -> (w718:u8)
        n225 = local write "Ring"(w709) -> ()
        n226 = Build Array(u8 75, w718, u8 4 ("Length"), u8 1, u8 0, u8 0, u8 0, u8 0) -> (→"packet PWM":u8[])
        n227 = local write "Time"("Plot Time") -> ()
        n228 = property on="Plot OFF" class="Bool"("Visible"=TRUE) -> ()  [unwired: 2 in, 2 out]
        n229 = property on="Plot On" class="Bool"("Visible"=FALSE) -> ()  [unwired: 2 in, 2 out]
        n230 = property on="Plot Time" class="DigNum (strict)"("Visible"=FALSE) -> ()  [unwired: 2 in, 2 out]
        "Time Plot" <- "Plot Time"
      }
      event "Plot OFF": Value Change {
        w728 = u16 0 items=["None", "Moment"] ("Ring")
        n231 = event-data() -> ()  [unwired: 1 in, 5 out]
        n232 = local write "Time"(200 ("Time")) -> ()
        n233 = local write "Ring"(w728) -> ()
        n234 = property on="Plot Time" class="DigNum (strict)"("Visible"=TRUE) -> ()  [unwired: 2 in, 2 out]
        n235 = property on="Plot OFF" class="Bool"("Visible"=FALSE) -> ()  [unwired: 2 in, 2 out]
        n236 = property on="Plot On" class="Bool"("Visible"=TRUE) -> ()  [unwired: 2 in, 2 out]
      }
      event "Clear": Value Change {
        n237 = event-data() -> ()  [unwired: 1 in, 5 out]
        n238 = Enqueue Element(queue=w735, element=u8[] [0, 0, 255, 69]) -> ()  [unwired: 1 in, 4 out]
      }
      event "stop": Value Change {
        w742 = TRUE ("Flag Stop R")
        n239 = event-data() -> ()  [unwired: 1 in, 5 out]
        n240 = VISA Close(VISA resource name=w740) -> (error out=→"error out":errorcluster)  [unwired: 1 in]
        n241 = local write "Flag Stop T"(w742) -> ()
        n242 = local write "Flag Stop R"(w742) -> ()
        n243 = local write "Flag Stop I"(w742) -> ()
        n244 = local write "Stop VI"(w742) -> ()
      }
      event "Disconect": Value Change {
        n245 = event-data() -> ()  [unwired: 1 in, 5 out]
        n246 = VISA Close(VISA resource name=w751) -> ()  [unwired: 1 in, 1 out]
      }
      event "Disconect 2": Value Change {
        n247 = event-data() -> ()  [unwired: 1 in, 5 out]
        n248 = VISA Close(VISA resource name=w754) -> ()  [unwired: 1 in, 1 out]
      }
      event Timeout {
        n249 = event-data() -> ()  [unwired: 1 in, 1 out]
        n250 = Not Equal?(x=w759, y=w760) -> (x != y?=w758:bool)
        n251 = And(x="Read On/Off", y=w758) -> (x .and. y?=w761:bool)
        n252 = case shown="True" w761 {
          tunnel: w759 -> [_ w770]
          frame False {
          }
          frame True {
            n253 = call "GetADCTester (SubVI) TesterLoop.vi"("GetADCTester"="GetADCTester", "TimeToGet"="TimeToGet", "VISA Refnum in"=w770) -> ("ADCValOutput Single"=→"ADCValOutput Single":dbl)  [unwired: 6 in, 2 out]
          }
        }
        n254 = case shown="0, Default" "Ring" {
          tunnel: [FALSE TRUE TRUE] -> w767
          tunnel: [u8[] [] ("packet PWM") w775 w777] -> w766
          frame 0, Default {
          }
          frame 1 {
            n255 = local read "packet PWM"() -> (w775:u8[])
          }
          frame 2 {
            n256 = local read "GetIO"() -> (w777:u8[])
          }
        }
      }
    }
    "status" <- w58
    "VISA" <- w59
    n257 = case shown="True" w62 {
      tunnel: w61 -> [_ w69]
      tunnel: w60 -> [_ w68]
      frame False {
      }
      frame True {
        n258 = flat-sequence {
          tunnel: w69 -> [w71]
          tunnel: [w71] -> w67
          tunnel: w68 -> [w72]
          tunnel: w67 -> [w73]
          frame #0 {
            n259 = Wait (ms)(milliseconds to wait=u32 10) -> ()  [unwired: 1 out]
          }
          frame #1 {
            n260 = Enqueue Element(queue=w73, element=w72) -> ()  [unwired: 1 in, 4 out]
          }
        }
      }
    }
    n261 = Wait (ms)(milliseconds to wait=u32 100) -> ()  [unwired: 1 out]
    n262 = Not(x=w58) -> (.not. x?=→"CommIcon":bool)
    n263 = Not(x=w52) -> (.not. x?=→"CommIcon Marvin":bool)
  }
  n264 = local write "RX"(w2) -> ()
  n265 = local write "TX"(w2) -> ()
  n266 = while {
    tunnel: w6 -> [w794]
    tunnel: errorcluster {"status"=FALSE, "code"=0, "source"=""} ("error out") -> [w793]
    tunnel: [w784] -> _
    tunnel: w28 -> [_]
    tunnel: [TRUE] -> _
    shift-right: [w789] -> _
    shift-left: w2 -> [w788]
    tunnel: w19 -> [w786]
    shift-right: [w780] -> _
    shift-left: w5 -> [w783]
    shift-right: [w781] -> _
    shift-left: w8 -> [w782]
    stop <- "Flag Stop I" stop-if-true
    # "Interpreter Task"
    n267 = Get Queue Status(queue=w794, error in (no error)=w793) -> (queue out=w792:refnum<queue>, error out=w787:errorcluster, # elements in queue=w785:i32)  [unwired: 6 out]
    "Int b" <- w785
    n268 = Wait (ms)(milliseconds to wait=u32 100) -> ()  [unwired: 1 out]
    n269 = case shown="0" w785 {
      tunnel: w792 -> [_ w813]
      tunnel: w787 -> [w799 w811]
      tunnel: [w799 w812] -> w784
      tunnel: [w798 w808] -> w789
      tunnel: w788 -> [w798 w810]
      tunnel: w786 -> [_ _]
      tunnel: w783 -> [w797 w803]
      tunnel: [w797 w800] -> w780
      tunnel: w782 -> [w796 w802]
      tunnel: [w796 w801] -> w781
      frame 0 {
        n270 = Wait (ms)(milliseconds to wait=u32 1) -> ()  [unwired: 1 out]
      }
      frame 1, Default {
        n271 = Dequeue Element(queue=w813, error in (no error)=w811) -> (element=w809:u8[], error out=w812:errorcluster)  [unwired: 3 out]
        "Read array" <- w809
        n272 = Index Array(array=w809, index #1=0 ("index")) -> (element #3=w805:u8)  [unwired: 2 in, 2 out]
        "Cmd Id" <- w805
        n273 = case shown="15..19" w805 {
          tunnel: w809 -> [_ w824 w849 w873 w903 w915 w929]
          tunnel: ["" w821 w848 w860 "" "" ""] -> w804
          tunnel: w803 -> [w815 w820 w843 w875 w905 w917 w931]
          tunnel: [w815 w819 w842 w875 w905 w917 w931] -> w800
          tunnel: w802 -> [w814 w818 w841 w874 w904 w916 w930]
          tunnel: [w814 w817 w838 w874 w904 w916 w930] -> w801
          frame 0, Default {
          }
          frame 255 {
            n274 = Index Array(array=w824, index=3) -> (element=w822:u8)
            n275 = case shown="69" w822 {
              tunnel: ["" "Clear Plot"] -> w821
              tunnel: [w827 cluster{"n":dbl, "T":dbl}[] [] ("Current Graph 4")] -> w819
              tunnel: w820 -> [w827 _]
              tunnel: w818 -> [w825 _]
              tunnel: [w825 u16 0 ("TempCnt")] -> w817
              frame 0, Default {
              }
              frame 69 {
              }
            }
          }
          frame 1 {
            # "y=1.9967x-19.97"
            n276 = Index Array(array=w849, index #1=3 ("index")) -> (element #1=w852:u8, element #2=w854:u8, element #3=w855:u8, element #4=w856:u8)  [unwired: 3 in]
            n277 = Join Numbers(hi=w856, lo=w855) -> ((hi.lo)=w850:u16)
            n278 = Join Numbers(hi=w854, lo=w852) -> ((hi.lo)=w851:u16)
            n279 = Join Numbers(hi=w850, lo=w851) -> ((hi.lo)=w847:u32)
            "PWM Reading" <- w847
            n280 = To Double Precision Float(number=w847) -> (double precision float=w846:dbl)
            n281 = Divide(x=w846, y=1000.0) -> (x/y=w835:dbl)
            "Frequency" <- w835
            n282 = Multiply(x=w835, y=1.9967) -> (x*y=w834:dbl)
            n283 = Subtract(x=w834, y=19.97) -> (x-y=w831:dbl)
            "Load" <- w831
            n284 = local read "Time Plot"() -> (w837:i32)
            n285 = Number To Fractional String(number=w831) -> (F-format string=w832:string)  [unwired: 3 in]
            n286 = Multiply(x=w837, y=w841) -> (x*y=w840:i32)
            n287 = Increment(x=w841) -> (x+1=w838:u16)
            n288 = To Double Precision Float(number=w840) -> (double precision float=w839:dbl)
            n289 = Bundle(w839, w831) -> (w844:cluster{dbl, dbl})  [unwired: 1 in]
            n290 = Build Array (concatenate)(w843, w844) -> (w842:cluster{"n":dbl, "T":dbl}[])
            n291 = Concatenate Strings("Load ", w832) -> (w848:string)
          }
          frame 10 {
            w859 = "." ("string")
            n292 = Index Array(array=w873, index #1=3 ("index")) -> (element #1=w869:u8, element #2=w872:u8, element #3=w871:u8, element #4=w870:u8)  [unwired: 3 in]
            n293 = Build Array(w869) -> (w868:u8[])
            n294 = Number To Decimal String(number=w872, width (-)=i16 2) -> (decimal integer string=w864:string)
            n295 = Byte Array To String(unsigned byte array=w868) -> (string=w858:string)
            n296 = Number To Decimal String(number=w871, width (-)=i16 2) -> (decimal integer string=w865:string)
            n297 = Number To Decimal String(number=w870, width (-)=i16 2) -> (decimal integer string=w867:string)
            n298 = Concatenate Strings("Version ", "  " ("string"), w867, w859, w865, w859, w864, w859, w858) -> (w860:string)
            "Ver" <- w860
          }
          frame 4 {
            n299 = Index Array(array=w903, index #1=3 ("index")) -> (element #1=w901:u8, element #2=w900:u8, element #3=w899:u8, element #4=w898:u8)  [unwired: 3 in]
            n300 = Join Numbers(hi=w900, lo=w901) -> ((hi.lo)=w897:u16)
            n301 = Join Numbers(hi=w898, lo=w899) -> ((hi.lo)=w896:u16)
            n302 = Join Numbers(hi=w896, lo=w897) -> ((hi.lo)=w895:u32)
            "(hi.lo)" <- w895
            n303 = Number To Boolean Array(number=w895) -> (Boolean array=w885:bool[])
            n304 = Index Array(array=w885, index #1=0 ("index")) -> (element #1=→"S1 GIO 1":bool, element #2=→"S2 GIO 18":bool, element #3=→"S2 GIO 19":bool, element #4=→"S1 GIO 19":bool, element #5=→"S1 GIO 18":bool, element #6=→"S1 GIO 17":bool, element #7=→"S1 GIO 15":bool)  [unwired: 6 in]
            n305 = Index Array(array=w885, index #1=7 ("index")) -> (element #1=→"S1 GIO 11":bool, element #2=→"S1 GIO 3":bool, element #3=→"S2 GIO 1":bool, element #4=→"S2 GIO 3":bool, element #5=→"S2 GIO 11":bool, element #6=→"S2 GIO 15 R":bool, element #7=→"S2 GIO 17":bool)  [unwired: 6 in]
          }
          frame 6 {
            n306 = Index Array(array=w915, index #1=3 ("index")) -> (element #1=w913:u8, element #2=w912:u8, element #3=w911:u8, element #4=w910:u8)  [unwired: 3 in]
            n307 = Join Numbers(hi=w912, lo=w913) -> ((hi.lo)=w909:u16)
            n308 = Join Numbers(hi=w910, lo=w911) -> ((hi.lo)=w908:u16)
            n309 = Join Numbers(hi=w908, lo=w909) -> ((hi.lo)=→"out_io1":u32)
          }
          frame 15..19 {
            n310 = Index Array(array=w929, index #1=3 ("index")) -> (element #1=w927:u8, element #2=w926:u8, element #3=w925:u8, element #4=w924:u8)  [unwired: 3 in]
            n311 = Join Numbers(hi=w926, lo=w927) -> ((hi.lo)=w923:u16)
            n312 = Join Numbers(hi=w924, lo=w925) -> ((hi.lo)=w922:u16)
            n313 = Join Numbers(hi=w922, lo=w923) -> ((hi.lo)=w921:u32)
            "out_io1 2" <- w921
            n314 = Multiply(x=0.0201416015625, y=w921) -> (x*y=→"x*y":dbl)
          }
        }
        "CurrSp Graph" <- w800
        n315 = call "CheckStr.vi"("String"=w804) -> ("s? t:f"=w806:string)
        n316 = Concatenate Strings(w806, w810) -> (w808:string)
        "String 2" <- w808
      }
    }
  }
  n317 = while {
    tunnel: [TRUE] -> _
    tunnel: w29 -> [_]
    tunnel: w6 -> [w943]
    tunnel: [w942] -> _
    tunnel: errorcluster {"status"=FALSE, "code"=0, "source"=""} -> [w941]
    shift-right: [w940] -> _
    shift-left: refnum<visa-resource-name> refnum ("Value") -> [w937]
    shift-right: [w938] -> _
    shift-left: FALSE ("Value") -> [w936]
    shift-right: [w939] -> _
    shift-left: FALSE ("Plot_T") -> [w935]
    tunnel: ["Flag Stop R"] -> _
    stop <- "Flag Stop R" stop-if-true
    # "Receive Task"
    n318 = case shown="False" w935 {
      tunnel: [w949 w951] -> w945
      tunnel: [w946 w950] -> w938
      tunnel: w937 -> [_ w951]
      tunnel: w936 -> [_ w950]
      frame False {
        n319 = control-ref of="VISA"() -> (w948:refnum<vi>)
        n320 = control-ref of="CommIcon"() -> (w947:refnum<vi>)
        n321 = property class="Bool (strict)"(reference=w947) -> ("Value"=w946:bool)  [unwired: 1 in, 2 out]
        n322 = property class="VISAName"(reference=w948) -> ("Value"=w949:refnum<visa-resource-name>)  [unwired: 1 in, 2 out]
      }
      frame True {
      }
    }
    n323 = Wait (ms)(milliseconds to wait=u32 100) -> ()  [unwired: 1 out]
    n324 = case shown="False" w938 {
      tunnel: w941 -> [w964 w1009]
      tunnel: w945 -> [w961 w1010]
      tunnel: [w953 w1010] -> w940
      tunnel: [w965 w1009] -> w942
      tunnel: w943 -> [w954 w1008]
      tunnel: [w966 w1008] -> _
      tunnel: [w963 FALSE ("Plot_T")] -> w939
      tunnel: w935 -> [w952 _]
      frame False {
        (unwired) u32 8 ("byte count")
        n325 = VISA Read(VISA resource name=w961, byte count=u32 1, error in (no error)=w964) -> (VISA resource name out=w956:refnum<visa-resource-name>, read buffer=w957:string, error out=w955:errorcluster)  [unwired: 1 out]
        n326 = String To Byte Array(string=w957) -> (unsigned byte array=w960:u8[])
        n327 = Index Array(array=w960, index=0) -> (element=w958:u8)
        n328 = case shown="75" w958 {
          tunnel: [w970 w988] -> w966
          tunnel: [w969 w987] -> w965
          tunnel: [FALSE w986] -> w963
          tunnel: w956 -> [w967 w982]
          tunnel: w955 -> [w969 w981]
          tunnel: w954 -> [w970 w974]
          tunnel: [w967 w973] -> w953
          tunnel: w952 -> [_ w972]
          frame 0, Default {
          }
          frame 75 {
            n329 = VISA Read(VISA resource name=w982, byte count=u32 3, error in (no error)=w981) -> (VISA resource name out=w977:refnum<visa-resource-name>, read buffer=w985:string, error out=w976:errorcluster)  [unwired: 1 out]
            n330 = String To Byte Array(string=w985) -> (unsigned byte array=w975:u8[])
            n331 = local read "Add Unit"() -> (w971:u8)
            n332 = Index Array(array=w975, index #1=0 ("index")) -> (element #1=w980:u8, element #2=w978:u8)  [unwired: 2 in, 1 out]
            n333 = Equal?(x=w971, y=w980) -> (x = y?=w979:bool)
            n334 = case shown="True" w979 {
              tunnel: [w992 w1005] -> w988
              tunnel: [w990 w1004] -> w987
              tunnel: [w989 w995] -> w986
              tunnel: w978 -> [_ w1003]
              tunnel: w977 -> [w991 w1002]
              tunnel: w976 -> [w990 w1001]
              tunnel: w975 -> [_ w999]
              tunnel: w974 -> [w992 w996]
              tunnel: [w991 w994] -> w973
              tunnel: w972 -> [w989 w995]
              frame False {
              }
              frame True {
                n335 = VISA Read(VISA resource name=w1002, byte count=w1003, error in (no error)=w1001) -> (VISA resource name out=w994:refnum<visa-resource-name>, read buffer=w993:string, error out=w1000:errorcluster)  [unwired: 1 out]
                "RX" <- w993
                n336 = String To Byte Array(string=w993) -> (unsigned byte array=w998:u8[])
                n337 = Insert Into Array(array=w999, new element=w998) -> (w997:u8[])  [unwired: 1 in]
                n338 = Enqueue Element(queue=w996, element=w997, error in (no error)=w1000) -> (queue out=w1005:refnum<queue>, error out=w1004:errorcluster)  [unwired: 2 out]
              }
            }
          }
        }
      }
      frame True {
        n339 = Wait (ms)(milliseconds to wait=u32 10) -> ()  [unwired: 1 out]
      }
    }
  }
  n340 = while {
    tunnel: w14 -> [_]
    tunnel: w13 -> [w1013]
    stop <- "Flag Stop T" stop-if-true
    # "Transmit task"
    n341 = control-ref of="VISA"() -> (w1017:refnum<vi>)
    n342 = control-ref of="CommIcon"() -> (w1018:refnum<vi>)
    n343 = property class="Bool (strict)"(reference=w1018) -> ("Value"=w1012:bool)  [unwired: 1 in, 2 out]
    n344 = property class="VISAName"(reference=w1017) -> ("Value"=w1016:refnum<visa-resource-name>)  [unwired: 1 in, 2 out]
    n345 = case shown="False" w1012 {
      tunnel: w1016 -> [w1020 _]
      tunnel: errorcluster {"status"=FALSE, "code"=0, "source"=""} -> [w1019 _]
      tunnel: w1013 -> [w1022 _]
      frame False {
        n346 = Get Queue Status(queue=w1022) -> (queue out=w1021:refnum<queue>, # elements in queue=w1023:i32)  [unwired: 1 in, 7 out]
        n347 = case shown="1, Default" w1023 {
          tunnel: w1021 -> [_ w1031]
          tunnel: w1020 -> [_ w1030]
          tunnel: w1019 -> [_ w1028]
          frame 0 {
            n348 = local write "TX"(FALSE ("TX")) -> ()
          }
          frame 1, Default {
            n349 = Dequeue Element(queue=w1031) -> (element=w1027:u8[])  [unwired: 1 in, 4 out]
            "Write array" <- w1027
            n350 = Byte Array To String(unsigned byte array=w1027) -> (string=w1025:string)
            "TX" <- w1025
            n351 = VISA Write(VISA resource name=w1030, write buffer=w1025, error in (no error)=w1028) -> (error out=→"err tx":errorcluster)  [unwired: 2 out]
            n352 = local write "TX"(TRUE ("TX")) -> ()
          }
        }
      }
      frame True {
        n353 = Wait (ms)(milliseconds to wait=u32 10) -> ()  [unwired: 1 out]
      }
    }
    n354 = Wait (ms)(milliseconds to wait=u32 100) -> ()  [unwired: 1 out]
  }
